vi "Recursive find VIs.vi"(8 "error in (no error)":errorcluster, 11 "Project Items":refnum<vi>[](array[refnum])) -> (0 "error out":errorcluster, 3 "VIs":set{path}(c389))   [LabVIEW 2020, in "Coverage Analyzer.lvclass"]
uses:
  Coverage Analyzer.lvclass
  Coverage Analyzer.lvclass/Coverage Analyzer.ctl
  a1401d1e-ec1c-4a27-9029-e4c0d22f2509.vi
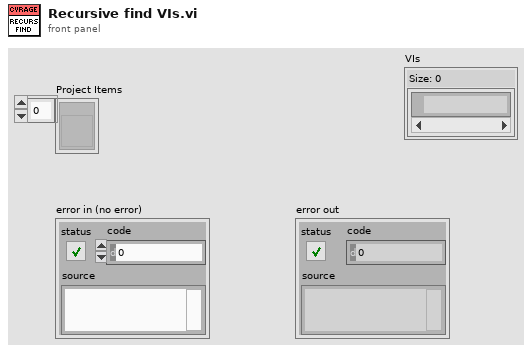
[diagram p1: front panel]
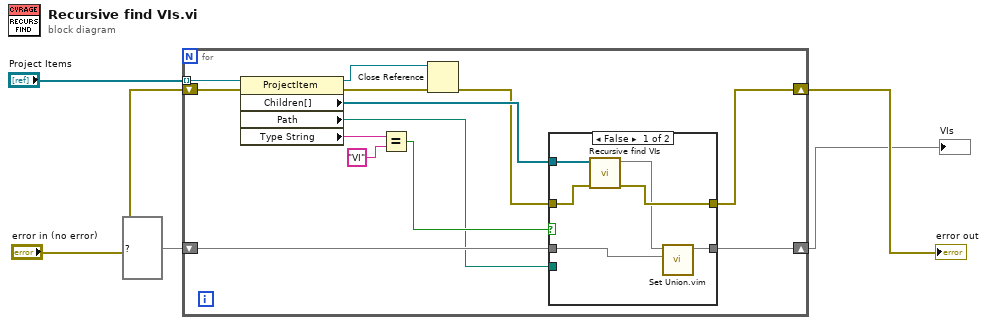
[diagram p0: block diagram]
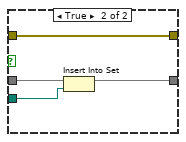
[diagram p2: hidden frame]
diagram:
  n1 = for {
    tunnel: "Project Items" -> [w15] mode=indexing
    shift-right: [w9] -> w3
    shift-left: "error in (no error)" -> [w14]
    shift-right: [w7] -> w1
    shift-left: set{path} {} ("VIs") -> [w8]
    n2 = property class="ProjectItem"(reference=w15, error in=w14) -> (reference out=w12:refnum<vi>, error out=w13:errorcluster, "Children[]"=w11:refnum<vi>[], "Path"=w6:path, "Type String"=w18:string)
    n3 = Equal?(x=w18, y="VI") -> (x = y?=w16:bool)
    n4 = Close Reference(reference=w12, error in (no error)=w13) -> (error out=w10:errorcluster)
    n5 = case shown="False" w16 {
      tunnel: w11 -> [w24 _]
      tunnel: [w19 w27] -> w7
      tunnel: w10 -> [w23 w28]
      tunnel: [w22 w28] -> w9
      tunnel: w8 -> [w20 w26]
      tunnel: w6 -> [_ w25]
      frame False {
        n6 = call "Recursive find VIs.vi"("error in (no error)"=w23, "Project Items"=w24) -> ("error out"=w22:errorcluster, "VIs"=w21:set{path})  [unwired: 8 in]
        n7 = call "Set Union.vim"("set 2"=w20, "set 1"=w21) -> ("union"=w19:set{path})  [unwired: 9 in]
      }
      frame True {
        n8 = Insert Into Set(10:w25, 11:w26) -> (3:w27:set{path})  [unwired: 1 out]
      }
    }
  }
  "error out" <- w3
  "VIs" <- w1
